vi "FA_ConvertToConfigData.vi"(8 "Error In":errorcluster, 11 "XML String":string) -> (0 "Error Out":errorcluster, 3 "ConfigData":T1)   [LabVIEW 2014, in "FA_NativeTypes.lvlib"]
doc: "Converts XML text describing a configuration to a LabVIEW cluster"
uses:
  FA_NativeTypes.lvlib
  FA_Config.ctl
  FA_LocalStore API/source/VI Source/FA_LSSpecialTypes.ctl
  FA_LocalStore API/source/VI Source/FA_LocalStore.lvlib
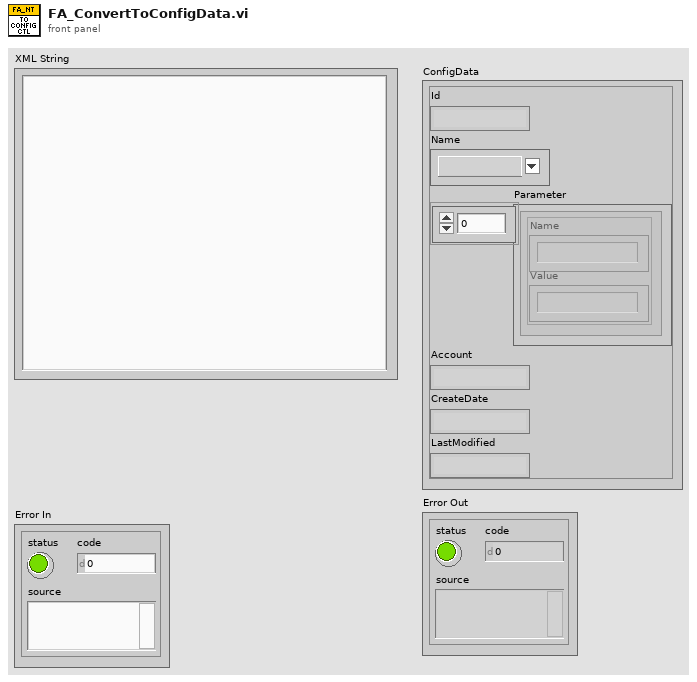
[diagram p1: front panel]
types:
  T1 = typedef "FA_NativeTypes.lvlib/FA_Config.ctl" = cluster{"Id":string, "Name":T2, "Parameter":cluster{"Name":string, "Value":string}[], "Account":string, "CreateDate":string, "LastModified":string}
  T2 = typedef "FA_LocalStore.lvlib/FA_LSSpecialTypes.ctl" = string
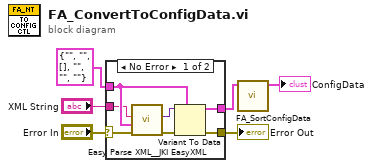
[diagram p0: block diagram]
diagram:
  n1 = case shown="No Error" "Error In" {
    selector: "Error In" -> [w13 w15]
    tunnel: [w8 w15] -> w5
    tunnel: T1 {"Id"="", "Name"="", "Parameter"=[], "Account"="", "CreateDate"="", "LastModified"=""} ("ConfigData") -> [w10 w14]
    tunnel: [w9 w14] -> w2
    tunnel: "XML String" -> [w7 _]
    frame No Error {
      n2 = call <vilib>:"Easy Parse XML__JKI EasyXML.vi"("error in (no error)"=w13, "LabVIEW Data (Type)"=w10, "XML String"=w7) -> ("error out"=w12:errorcluster, "LabVIEW Data"=w11:variant)  [unwired: 7 in]
      n3 = Variant To Data(error in=w12, type=w10, Variant=w11) -> (data=w9:T1, error out=w8:errorcluster)
    }
    frame Error {
    }
  }
  "Error Out" <- w5
  n4 = call "FA_SortConfigData.vi"("Config In"=w2) -> ("Config"=→"ConfigData":T1)  [unwired: 10 in]
